vi "InitializePWM.vi"() -> (0 "Motor PWMs":T8)   [LabVIEW 2018]
uses:
  <vilib>/myRIO/Instrument Drivers/Onboard IO/PWM/typedefs/PWM Reference.ctl
  <vilib>/myRIO/Common/Instrument Driver Framework/Utilities/typedefs/myRIO Generic Hardware Reference.ctl
  <vilib>/myRIO/Common/Instrument Driver Framework/Utilities/typedefs/Hardware Version Enum.ctl
  <vilib>/myRIO/Common/Instrument Driver Framework/Utilities/typedefs/myRIO v1.0 Reference.ctl
  <vilib>/myRIO/Common/Instrument Driver Framework/Utilities/typedefs/Generic FPGA Reference.ctl
  <vilib>/myRIO/Common/Instrument Driver Framework/myRIO v1.0/PWM/typedefs/PWM Channels Enum.ctl
  <vilib>/myRIO/Instrument Drivers/Onboard IO/PWM/typedefs/PWM Configuration.ctl
  <vilib>/userdefined/High Color/nirio_resource_hc.ctl
  <vilib>/myRIO/Common/Instrument Driver Framework/myRIO v1.0/PWM/vis/myRIO v1.1 Open PWM.vi
  <vilib>/myRIO/Common/Instrument Driver Framework/Utilities/vis/Validate Channels.vi
  <vilib>/myRIO/Common/Instrument Driver Framework/myRIO v1.0/PWM/vis/myRIO v1.0 Reserve PWM.vi
  <vilib>/myRIO/Common/Instrument Driver Framework/myRIO v1.0/PWM/vis/myRIO v1.0 Build MUX Configuration PWM.vi
  <vilib>/myRIO/Common/Instrument Driver Framework/myRIO v1.0/Resource Manager/vis/myRIO v1.0 Reserve Channel List.vi
  <vilib>/myRIO/Common/Instrument Driver Framework/myRIO v1.0/Resource Manager/vis/myRIO v1.0 Create Configuration List.vi
  <vilib>/myRIO/Common/Instrument Driver Framework/myRIO v1.0/Resource Manager/vis/myRIO v1.0 Reserve Channel.vi
  <vilib>/myRIO/Common/Instrument Driver Framework/myRIO v1.0/Resource Manager/vis/myRIO v1.0 Unreserve Channel.vi
  <vilib>/myRIO/Common/Instrument Driver Framework/myRIO v1.0/Resource Manager/vis/myRIO v1.0 Build Mutex Name.vi
  <vilib>/Utility/VariantDataType/GetNumericInfo.vi
  <vilib>/Utility/error.llb/Error Cluster From Error Code.vi
  <vilib>/myRIO/Common/Instrument Driver Framework/myRIO v1.0/myRIO v1.1 Open.vi
  <vilib>/myRIO/Common/Instrument Driver Framework/Utilities/vis/IO Manager.vi
  <vilib>/myRIO/Common/Instrument Driver Framework/Utilities/vis/Configuration Manager.vi
  <vilib>/myRIO/Common/Instrument Driver Framework/myRIO v1.0/Resource Manager/vis/myRIO v1.0 Configure IO.vi
  <vilib>/myRIO/Common/Instrument Driver Framework/myRIO v1.0/myRIO v1.0 Close.vi
  <vilib>/myRIO/Common/Instrument Driver Framework/myRIO v1.0/PWM/vis/myRIO v1.0 Write PWM.vi
  <vilib>/myRIO/Instrument Drivers/Onboard IO/PWM/vis/myRIO PWM Open.xnode
  <vilib>/myRIO/Instrument Drivers/Onboard IO/PWM/PWM.lvlib
panel:
  # "This Vi initializes the PWM outputs on the myRIO so that they can drive the motors"
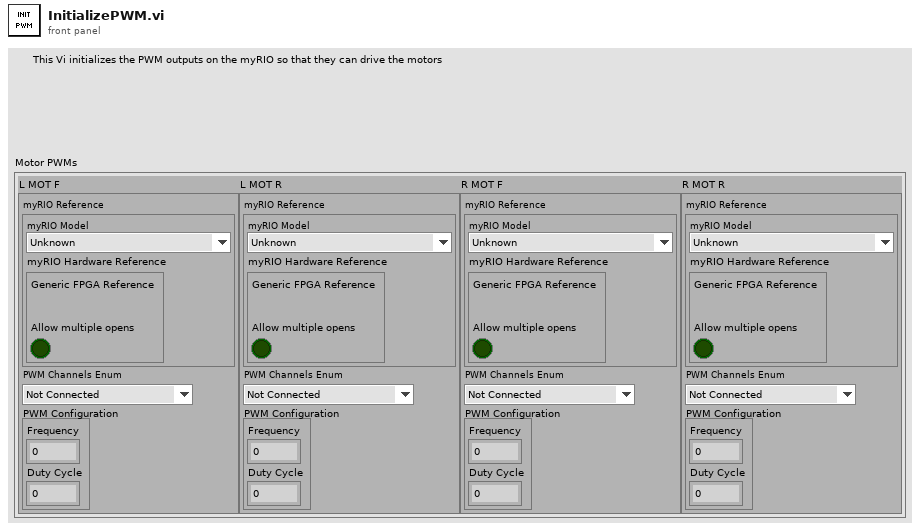
[diagram p1: front panel]
types:
  T1 = typedef "PWM.lvlib/PWM Reference.ctl" = cluster{"myRIO Reference":T2, "PWM Channels Enum":T6, "PWM Configuration":T7}
  T2 = typedef "myRIO Generic Hardware Reference.ctl" = cluster{"myRIO Model":T3, "myRIO Hardware Reference":T4}
  T3 = typedef "Hardware Version Enum.ctl" = enum16{"Unknown", "myRIO-1900", "myRIO-1950", "roboRIO", "NI ELVIS RIO CM", "ELVIS III"}
  T4 = typedef "myRIO v1.0 Reference.ctl" = cluster{"Generic FPGA Reference":T5, "Allow multiple opens":bool}
  T5 = typedef "Generic FPGA Reference.ctl" = refnum<k20>
  T6 = typedef "PWM Channels Enum.ctl" = enum16{"Not Connected", "C/PWM0", "C/PWM1", "A/PWM0", "A/PWM1", "A/PWM2", "A/PWM3", "A/PWM4", "A/PWM5", "A/PWM6", "A/PWM7", "A/PWM8", "A/PWM9", "A/PWM10", "A/PWM11", "A/PWM12", "A/PWM13", "A/PWM14", "A/PWM15", "A/PWM16", "A/PWM17", "A/PWM18", "A/PWM19", "B/PWM0", "B/PWM1", "B/PWM2", "B/PWM3", "B/PWM4", "B/PWM5", "B/PWM6", "B/PWM7", "B/PWM8", "B/PWM9", "B/PWM10", "B/PWM11", "B/PWM12", "B/PWM13", "B/PWM14", "B/PWM15", "B/PWM16", "B/PWM17", "B/PWM18", "B/PWM19", "PWM/PWM0", "PWM/PWM1", "PWM/PWM2", "PWM/PWM3", "PWM/PWM4", "PWM/PWM5", "PWM/PWM6", "PWM/PWM7", "PWM/PWM8", "PWM/PWM9"}
  T7 = typedef "PWM.lvlib/PWM Configuration.ctl" = cluster{"Frequency":dbl, "Duty Cycle":dbl}
  T8 = cluster{"L MOT F ":T1, "L MOT R":T1, "R MOT F":T1, "R MOT R":T1}
  T9 = cluster{"PWM Ref Out":T1, "PWM Ref Out":T1, "PWM Ref Out":T1, "PWM Ref Out":T1}
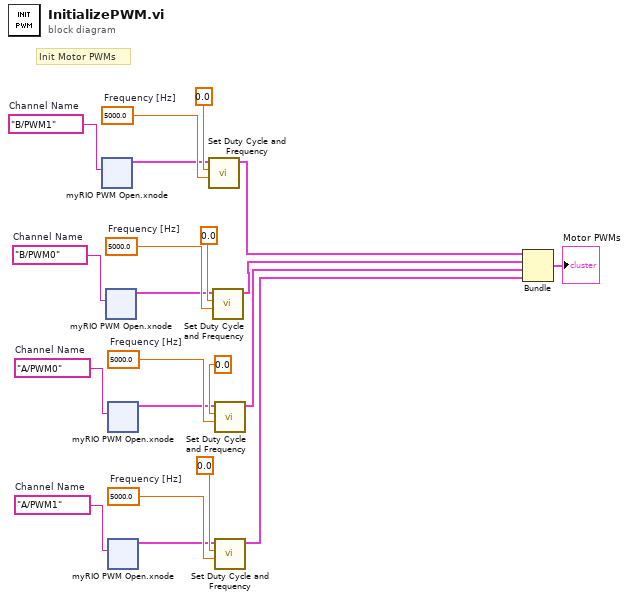
[diagram p0: block diagram]
diagram:
  w7 = 5000.0  # Frequency [Hz]
  w9 = tag "A/PWM1"  # Channel Name
  w11 = 5000.0  # Frequency [Hz]
  w13 = tag "A/PWM0"  # Channel Name
  w16 = 5000.0  # Frequency [Hz]
  w18 = tag "B/PWM0"  # Channel Name
  w19 = 5000.0  # Frequency [Hz]
  w21 = tag "B/PWM1"  # Channel Name
  # "Init Motor PWMs"
  n1 = xnode "myRIO PWM Open.xnode"("Channel Name"=w21) -> ("PWM Ref Out"=w14:T1)  [unwired: 2 in, 1 out]
  n2 = xnode "myRIO PWM Open.xnode"("Channel Name"=w18) -> ("PWM Ref Out"=w15:T1)  [unwired: 2 in, 1 out]
  n3 = xnode "myRIO PWM Open.xnode"("Channel Name"=w13) -> ("PWM Ref Out"=w10:T1)  [unwired: 2 in, 1 out]
  n4 = xnode "myRIO PWM Open.xnode"("Channel Name"=w9) -> ("PWM Ref Out"=w6:T1)  [unwired: 2 in, 1 out]
  n5 = call <vilib>:"Set Duty Cycle and Frequency.vi"("Frequency [Hz]"=w19, "Duty Cycle"=0.0, "PWM Ref In"=w14) -> ("PWM Ref Out"=w5:T1)  [unwired: 6 in, 1 out]
  n6 = call <vilib>:"Set Duty Cycle and Frequency.vi"("Frequency [Hz]"=w16, "Duty Cycle"=0.0, "PWM Ref In"=w15) -> ("PWM Ref Out"=w4:T1)  [unwired: 6 in, 1 out]
  n7 = call <vilib>:"Set Duty Cycle and Frequency.vi"("Frequency [Hz]"=w11, "Duty Cycle"=0.0, "PWM Ref In"=w10) -> ("PWM Ref Out"=w3:T1)  [unwired: 6 in, 1 out]
  n8 = call <vilib>:"Set Duty Cycle and Frequency.vi"("Frequency [Hz]"=w7, "Duty Cycle"=0.0, "PWM Ref In"=w6) -> ("PWM Ref Out"=w2:T1)  [unwired: 6 in, 1 out]
  n9 = Bundle("PWM Ref Out"=w5, "PWM Ref Out"=w4, "PWM Ref Out"=w3, "PWM Ref Out"=w2) -> (→"Motor PWMs":T9)  [unwired: 1 in]
